vi "MAX31855USB_top.vi"() -> ()   [LabVIEW 2014]
panel:
  out "Channel 3":dbl format="%_4f °C"
  out "Channel 2":dbl format="%_4f °C"
  out "Channel 1":dbl format="%_4f °C"
  out "Channel 0":dbl format="%_4f °C"
  in  "Stopp":bool
  in  "Serial Configuration":T1={"Baud Rate"=9600, "Parity"=0, "Data Bits"=8, "Stop Bits"=10, "Flow Control"=0} {"Flow Control" items=["None", "XON/XOFF", "RTS/CTS", "XON/XOFF & RTS/CTS", "DTR/DSR", "XON/XOFF & DTR/DSR"]; "Stop Bits" items=["1.0"=10, "1.5"=15, "2.0"=20]; "Data Bits" items=["7"=7, "8"=8]; "Parity" items=["None", "Odd", "Even", "Mark", "Space"]; "Baud Rate" items=["300"=300, "600"=600, "1200"=1200, "2400"=2400, "4800"=4800, "9600"=9600, "19200"=19200]}
  in  "VISA resource name":refnum<visa-resource-name>
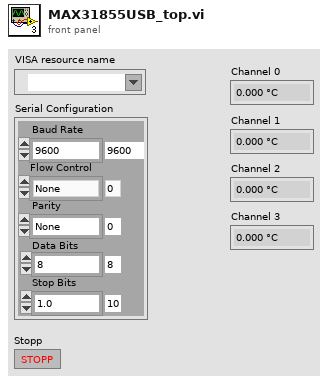
[diagram p1: front panel]
types:
  T1 = cluster{"Baud Rate":u32, "Parity":u16, "Data Bits":u16, "Stop Bits":u16, "Flow Control":u16}
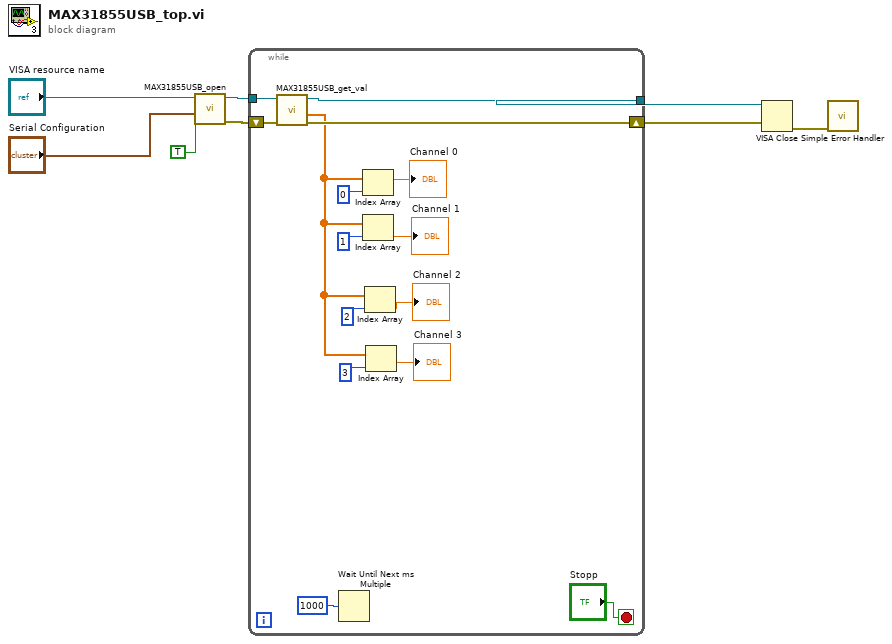
[diagram p0: block diagram]
diagram:
  n1 = call "MAX31855USB_open.vi"("Serial Configuration"="Serial Configuration", "ID Query (True)"=TRUE, "VISA resource name"="VISA resource name") -> ("error out"=w1:errorcluster, "VISA resource name out"=w2:refnum<visa-resource-name>)  [unwired: 7 in]
  n2 = while {
    tunnel: w2 -> [w21]
    shift-right: [w18] -> w8
    shift-left: w1 -> [w20]
    tunnel: [w19] -> w7
    stop <- "Stopp" stop-if-true
    n3 = call "MAX31855USB_get_val.vi"("error in (no error)"=w20, "VISA resource name"=w21) -> ("error out"=w18:errorcluster, "array"=w9:dbl[], "VISA resource name out"=w19:refnum<visa-resource-name>)  [unwired: 3 in]
    n4 = Wait Until Next ms Multiple(millisecond multiple=u32 1000 ("ms")) -> ()  [unwired: 1 out]
    n5 = Index Array(array=w9, index=0) -> (element=→"Channel 0":dbl)
    n6 = Index Array(array=w9, index=1) -> (element=→"Channel 1":dbl)
    n7 = Index Array(array=w9, index=2) -> (element=→"Channel 2":dbl)
    n8 = Index Array(array=w9, index=3) -> (element=→"Channel 3":dbl)
  }
  n9 = VISA Close(VISA resource name=w7, error in (no error)=w8) -> (error out=w6:errorcluster)
  n10 = call <vilib>:"Simple Error Handler.vi"("error in (no error)"=w6) -> ()  [unwired: 4 in, 5 out]
